vi "Impedance_Single_Meas.vi"(0 "frequency":dbl=10000.0 format="%#.2p", 1 "Time":dbl=0.05 format="%#_6p", 3 "SampRate":dbl=250000.0 format="%#.3p", 5 "Output channels":tag="Dev3/ao0", 9 "Voltage Ch":tag="Dev3/ai0", 11 "Current Ch":tag="Dev3/ai1", 12 "TriggerLine":tag="/Dev3/ao/StartTrigger", 14 "amplitude":dbl=0.1 format="%#.3p") -> (4 "Time domain Voltage":waveform(dbl)(graph)={"t0"=timestamp(3723563003.6430054 s since 1904-01-01), "dt"=3.999999999999989e-06, "Y"=array[12500 elements], "attributes"=variant("NI_ChannelName"=variant(string "Dev3/ai0"), "NI_UnitDescription"=variant(string "Volts"))}, 6 "Time domain Current":waveform(dbl)(graph)={"t0"=timestamp(3723563003.771688 s since 1904-01-01), "dt"=3.999999999999989e-06, "Y"=array[12500 elements], "attributes"=variant("NI_ChannelName"=variant(string "Dev3/ai1"), "NI_UnitDescription"=variant(string "Volts"))}, 10 "Voltage Complex":cdb=0.02528247639303564+0.006352558786407083i, 15 "Current Complex":cdb=1.0329648792920967-0.39524749923610863i)   [LabVIEW 2020]
uses:
  <vilib>/DAQmx/write.llb/DAQmx Write (Analog Wfm 1Chan NSamp).vi
  <vilib>/DAQmx/read.llb/DAQmx Read (Analog 1D Wfm NChan NSamp).vi
  <vilib>/DAQmx/create/channels.llb/DAQmx Create Channel (AO-Voltage-Basic).vi
  <vilib>/DAQmx/create/channels.llb/DAQmx Create Channel (AI-Voltage-Basic).vi
  <vilib>/DAQmx/configure/timing.llb/DAQmx Timing (Sample Clock).vi
  <vilib>/DAQmx/miscellaneous.llb/DAQmx Fill In Error Info.vi
  <vilib>/DAQmx/configure/trigger.llb/DAQmx Start Trigger (Digital Edge).vi
  <vilib>/measure/matone.llb/Extract Single Tone Information 1 Chan.vi
  <vilib>/measure/NI_MABase.lvlib
  <vilib>/measure/NI_MAPro.lvlib
panel:
  out "Time domain Current 2":waveform(dbl)(graph)={"t0"=timestamp(3723563003.771688 s since 1904-01-01), "dt"=3.999999999999989e-06, "Y"=array[12500 elements], "attributes"=variant("NI_ChannelName"=variant(string "Dev3/ai1"), "NI_UnitDescription"=variant(string "Volts"))}
  out "Time domain Voltage 2":waveform(dbl)(graph)={"t0"=timestamp(3723563003.6430054 s since 1904-01-01), "dt"=3.999999999999989e-06, "Y"=array[12500 elements], "attributes"=variant("NI_ChannelName"=variant(string "Dev3/ai0"), "NI_UnitDescription"=variant(string "Volts"))}
  out "detected frequency 2":dbl format="%.2p"
  out "detected frequency":dbl format="%.2p"
  out "Current phase (deg)":dbl=-20.938550713462377 format="%.2p"
  out "Voltage phase (deg)":dbl=14.104347915620849 format="%.2p"
  in  "CurentRangeMax":dbl=5.0 format="%0.2f"
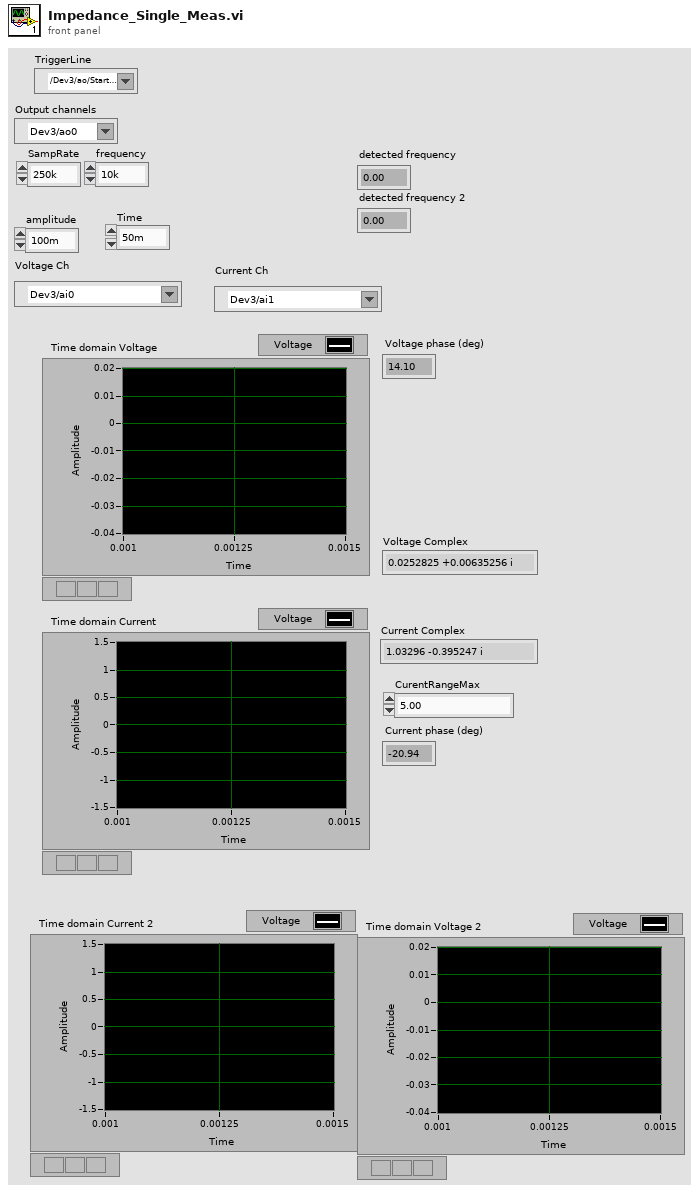
[diagram p1: front panel]
types:
  T1 = enum32{"none", "input signal", "detected signal", "residual signal"}
  T2 = cluster{"exported time signal":waveform(dbl), "exported spectrum (dB)":cluster{"f0":dbl, "df":dbl, "dB Spectrum (Hann)":dbl[]}}
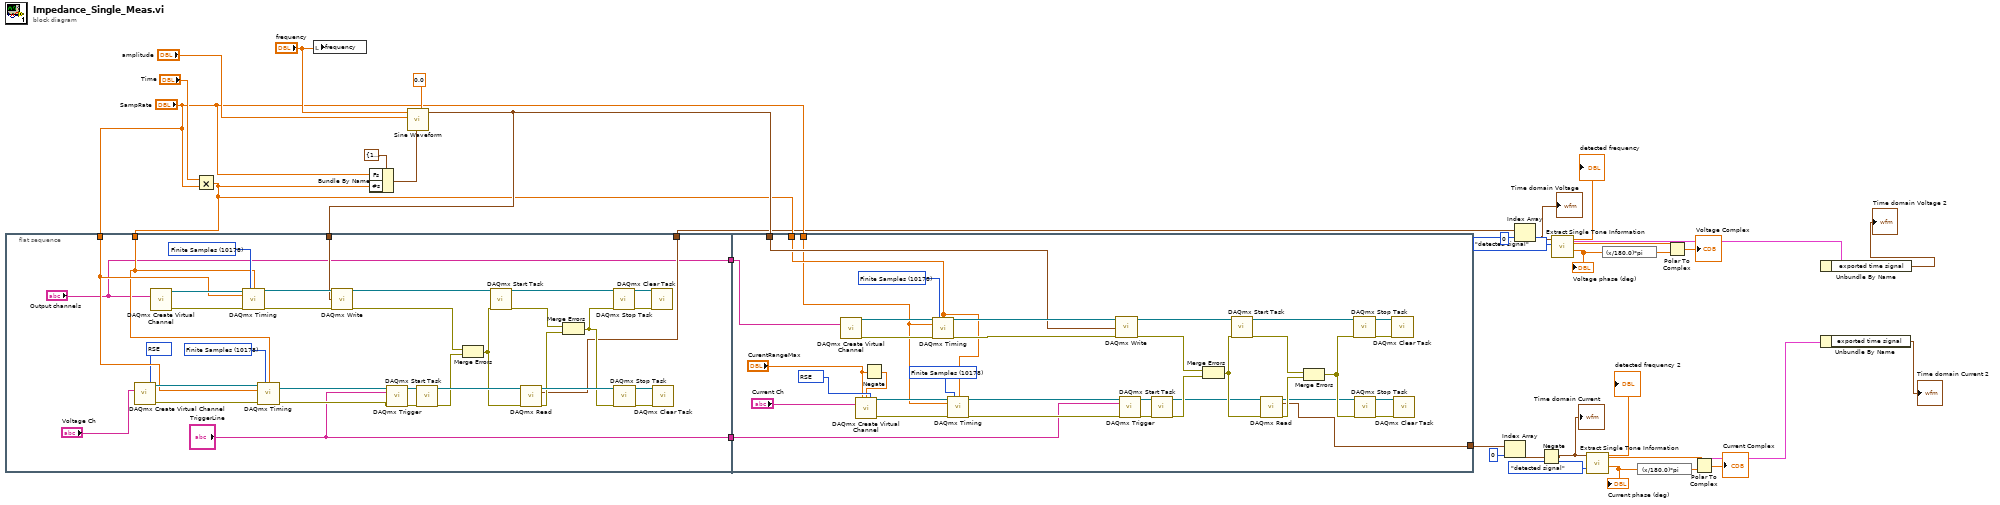
[diagram p0: block diagram]
diagram:
  n1 = flat-sequence {
    tunnel: "SampRate" -> [w45]
    tunnel: w26 -> [w44]
    tunnel: w27 -> [w42]
    tunnel: [w37] -> w21
    tunnel: ["Output channels"] -> w28
    tunnel: ["TriggerLine"] -> w1
    tunnel: w28 -> [w76]
    tunnel: [w75] -> w15
    tunnel: w27 -> [w74]
    tunnel: w26 -> [w73]
    tunnel: "SampRate" -> [w72]
    tunnel: w1 -> [w69]
    frame #0 {
      w43 = 10083 items=["Default"=-1, "RSE"=10083, "NRSE"=10078, "Differential"=10106, "Pseudodifferential"=12529] ("input terminal configuration")
      w57 = 10178 items=["Finite Samples"=10178, "Continuous Samples"=10123, "Hardware Timed Single Point"=12522] ("sample mode")
      w61 = 10178 items=["Finite Samples"=10178, "Continuous Samples"=10123, "Hardware Timed Single Point"=12522] ("sample mode")
      n2 = call-poly <vilib>:"DAQmx Create Virtual Channel.vi"("input terminal configuration"=w43, "physical channels"="Voltage Ch") -> ("task out"=w59:refnum<k21>, "error out"=w60:errorcluster)  [unwired: 12 in]
      n3 = call-poly <vilib>:"DAQmx Create Virtual Channel.vi"("physical channels"="Output channels") -> ("task out"=w68:refnum<k21>, "error out"=w64:errorcluster)  [unwired: 13 in]
      n4 = call-poly <vilib>:"DAQmx Timing.vi"("task/channels in"=w68, "sample mode"=w61, "samples per channel"=w44, "rate"=w45, "error in"=w64) -> ("task out"=w67:refnum<k21>, "error out"=w65:errorcluster)  [unwired: 9 in]
      n5 = call-poly <vilib>:"DAQmx Timing.vi"("task/channels in"=w59, "sample mode"=w57, "samples per channel"=w44, "rate"=w45, "error in"=w60) -> ("task out"=w56:refnum<k21>, "error out"=w55:errorcluster)  [unwired: 9 in]
      n6 = call-poly <vilib>:"DAQmx Write.vi"("task/channels in"=w67, "data"=w42, "error in"=w65) -> ("task out"=w66:refnum<k21>, "error out"=w47:errorcluster)  [unwired: 10 in, 1 out]
      n7 = call-poly <vilib>:"DAQmx Trigger.vi"("task/channels in"=w56, "source"="TriggerLine", "error in"=w55) -> ("task out"=w53:refnum<k21>, "error out"=w54:errorcluster)  [unwired: 11 in]
      n8 = call <vilib>:"DAQmx Start Task.vi"("task/channels in"=w53, "error in"=w54) -> ("task out"=w52:refnum<k21>, "error out"=w48:errorcluster)  [unwired: 12 in]
      n9 = Merge Errors(w47, w48) -> (w46:errorcluster)
      n10 = call <vilib>:"DAQmx Start Task.vi"("task/channels in"=w66, "error in"=w46) -> ("task out"=w63:refnum<k21>, "error out"=w39:errorcluster)  [unwired: 12 in]
      n11 = call-poly <vilib>:"DAQmx Read.vi"("task/channels in"=w52, "error in"=w46) -> ("task out"=w49:refnum<k21>, "data"=w37:waveform(dbl)[], "error out"=w40:errorcluster)  [unwired: 11 in]
      n12 = Merge Errors(w39, w40) -> (w38:errorcluster)
      n13 = call <vilib>:"DAQmx Stop Task.vi"("task/channels in"=w63, "error in"=w38) -> ("task out"=w62:refnum<k21>, "error out"=w41:errorcluster)  [unwired: 12 in]
      n14 = call <vilib>:"DAQmx Stop Task.vi"("task/channels in"=w49, "error in"=w38) -> ("task out"=w50:refnum<k21>, "error out"=w51:errorcluster)  [unwired: 12 in]
      n15 = call <vilib>:"DAQmx Clear Task.vi"("task in"=w62, "error in"=w41) -> ()  [unwired: 13 in, 1 out]
      n16 = call <vilib>:"DAQmx Clear Task.vi"("task in"=w50, "error in"=w51) -> ()  [unwired: 13 in, 1 out]
    }
    frame #1 {
      w100 = 10083 items=["Default"=-1, "RSE"=10083, "NRSE"=10078, "Differential"=10106, "Pseudodifferential"=12529] ("input terminal configuration")
      w88 = 10178 items=["Finite Samples"=10178, "Continuous Samples"=10123, "Hardware Timed Single Point"=12522] ("sample mode")
      w84 = 10178 items=["Finite Samples"=10178, "Continuous Samples"=10123, "Hardware Timed Single Point"=12522] ("sample mode")
      n17 = call-poly <vilib>:"DAQmx Create Virtual Channel.vi"("physical channels"=w76) -> ("task out"=w77:refnum<k21>, "error out"=w81:errorcluster)  [unwired: 13 in]
      n18 = Negate(x="CurentRangeMax") -> (-x=w70:dbl)
      n19 = call-poly <vilib>:"DAQmx Create Virtual Channel.vi"("maximum value"="CurentRangeMax", "minimum value"=w70, "input terminal configuration"=w100, "physical channels"="Current Ch") -> ("task out"=w86:refnum<k21>, "error out"=w85:errorcluster)  [unwired: 10 in]
      n20 = call-poly <vilib>:"DAQmx Timing.vi"("task/channels in"=w77, "sample mode"=w84, "samples per channel"=w73, "rate"=w72, "error in"=w81) -> ("task out"=w78:refnum<k21>, "error out"=w80:errorcluster)  [unwired: 9 in]
      n21 = call-poly <vilib>:"DAQmx Timing.vi"("task/channels in"=w86, "sample mode"=w88, "samples per channel"=w73, "rate"=w72, "error in"=w85) -> ("task out"=w89:refnum<k21>, "error out"=w90:errorcluster)  [unwired: 9 in]
      n22 = call-poly <vilib>:"DAQmx Write.vi"("task/channels in"=w78, "data"=w74, "error in"=w80) -> ("task out"=w79:refnum<k21>, "error out"=w98:errorcluster)  [unwired: 10 in, 1 out]
      n23 = call-poly <vilib>:"DAQmx Trigger.vi"("task/channels in"=w89, "source"=w69, "error in"=w90) -> ("task out"=w92:refnum<k21>, "error out"=w91:errorcluster)  [unwired: 11 in]
      n24 = call <vilib>:"DAQmx Start Task.vi"("task/channels in"=w92, "error in"=w91) -> ("task out"=w93:refnum<k21>, "error out"=w97:errorcluster)  [unwired: 12 in]
      n25 = Merge Errors(w98, w97) -> (w99:errorcluster)
      n26 = call <vilib>:"DAQmx Start Task.vi"("task/channels in"=w79, "error in"=w99) -> ("task out"=w82:refnum<k21>, "error out"=w103:errorcluster)  [unwired: 12 in]
      n27 = call-poly <vilib>:"DAQmx Read.vi"("task/channels in"=w93, "error in"=w99) -> ("task out"=w96:refnum<k21>, "data"=w75:waveform(dbl)[], "error out"=w102:errorcluster)  [unwired: 11 in]
      n28 = Merge Errors(w103, w102) -> (w104:errorcluster)
      n29 = call <vilib>:"DAQmx Stop Task.vi"("task/channels in"=w82, "error in"=w104) -> ("task out"=w83:refnum<k21>, "error out"=w101:errorcluster)  [unwired: 12 in]
      n30 = call <vilib>:"DAQmx Stop Task.vi"("task/channels in"=w96, "error in"=w104) -> ("task out"=w95:refnum<k21>, "error out"=w94:errorcluster)  [unwired: 12 in]
      n31 = call <vilib>:"DAQmx Clear Task.vi"("task in"=w83, "error in"=w101) -> ()  [unwired: 13 in, 1 out]
      n32 = call <vilib>:"DAQmx Clear Task.vi"("task in"=w95, "error in"=w94) -> ()  [unwired: 13 in, 1 out]
    }
  }
  n33 = Multiply(x="Time", y="SampRate") -> (x*y=w26:dbl)
  n34 = local write "frequency"("frequency") -> ()
  n35 = Bundle By Name(cluster=cluster{"Fs":dbl, "#s":dbl} {"Fs"=1000.0, "#s"=1000.0} ("sampling info"), "Fs"="SampRate", "#s"=w26) -> (w30:cluster{"Fs":dbl, "#s":dbl})
  n36 = call <vilib>:"Sine Waveform.vi"("offset"=0.0, "sampling info"=w30, "amplitude"="amplitude", "frequency"="frequency") -> ("signal out"=w27:waveform(dbl))  [unwired: 6 in, 1 out]
  n37 = Index Array(array=w15, index=0) -> (element=w10:waveform(dbl))
  n38 = Index Array(array=w21, index=0) -> (element=w12:waveform(dbl))
  "Time domain Voltage" <- w12
  n39 = Negate(x=w10) -> (-x=w11:waveform(dbl))
  "Time domain Current" <- w11
  n40 = call-poly <vilib>:"Extract Single Tone Information.vi"("export mode"=T1."detected signal", "time signal in"=w12) -> ("detected phase (deg)"=w23:dbl, "detected amplitude"=w24:dbl, "detected frequency"=→"detected frequency":dbl, "exported signals"=w5:T2)  [unwired: 4 in, 2 out]
  "Voltage phase (deg)" <- w23
  n41 = call-poly <vilib>:"Extract Single Tone Information.vi"("export mode"=T1."detected signal", "time signal in"=w11) -> ("detected phase (deg)"=w18:dbl, "detected amplitude"=w19:dbl, "detected frequency"=→"detected frequency 2":dbl, "exported signals"=w4:T2)  [unwired: 4 in, 2 out]
  "Current phase (deg)" <- w18
  n42 = expression code="(x/180.0)*pi" ("degrees to radians")(w23) -> (w22:dbl)
  n43 = expression code="(x/180.0)*pi" ("degrees to radians")(w18) -> (w17:dbl)
  n44 = Polar To Complex(1:w22, 2:w24) -> (0:→"Voltage Complex":cdb)
  n45 = Polar To Complex(1:w17, 2:w19) -> (0:→"Current Complex":cdb)
  n46 = Unbundle By Name(w4) -> ("exported time signal"=→"Time domain Current 2":waveform(dbl))
  n47 = Unbundle By Name(w5) -> ("exported time signal"=→"Time domain Voltage 2":waveform(dbl))
